vi "Adjust FP VI.vi"(8 "error in (no error)":errorcluster, 11 "QD Launch VI Ref":refnum<vi>) -> (0 "error out":errorcluster)   [LabVIEW 2023, in "Adjust FP VIs.lvlib"]
doc: "Adjust FP VIs"
uses:
  Adjust FP VIs.lvlib
panel:
  in  "Undo Name":string="Arrange VI Window"
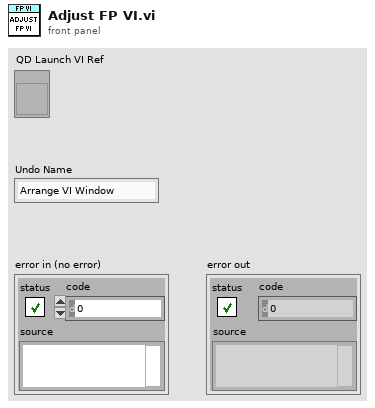
[diagram p1: front panel]
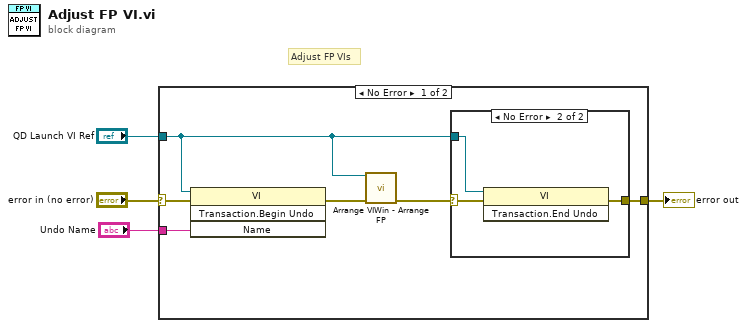
[diagram p0: block diagram]
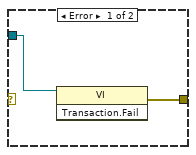
[diagram p2: hidden frame]
diagram:
  # "Adjust FP VIs"
  n1 = case shown="No Error" "error in (no error)" {
    selector: "error in (no error)" -> [w9 w16]
    tunnel: [w10 w16] -> w3
    tunnel: "QD Launch VI Ref" -> [w8 _]
    tunnel: "Undo Name" -> [w7 _]
    frame No Error {
      n2 = invoke class="VI" method="Transaction.Begin Undo"(reference=w8, error in=w9, "Name"=w7) -> (error out=w6:errorcluster)  [unwired: 1 in, 3 out]
      n3 = call <resource>:"Arrange VIWin - Arrange FP.vi"("VI"=w8, "error in"=w6) -> ("error out"=w5:errorcluster)  [unwired: 13 in]
      n4 = case shown="No Error" w5 {
        selector: w5 -> [_ w13]
        tunnel: w8 -> [w11 w14]
        tunnel: [w12 w15] -> w10
        frame Error {
          n5 = invoke class="VI" method="Transaction.Fail"(reference=w11) -> (error out=w12:errorcluster)  [unwired: 2 in, 2 out]
        }
        frame No Error {
          n6 = invoke class="VI" method="Transaction.End Undo"(reference=w14, error in=w13) -> (error out=w15:errorcluster)  [unwired: 1 in, 2 out]
        }
      }
    }
    frame Error {
    }
  }
  "error out" <- w3
